vi "Init_core.vi"(8 "error in (no error)":errorcluster, 10 "VIRefIn":refnum<vi>, 11 "CtlReferences in":refnum<class "CtlReferences.lvclass">) -> (0 "error out":errorcluster, 3 "CtlReferences out":refnum<class "CtlReferences.lvclass">)   [LabVIEW 2020, in "CtlReferences.lvlib" / "CtlReferences.lvclass"]
uses:
  CtlReferences.lvclass
  CtlReferences.lvclass/CtlReferences.ctl
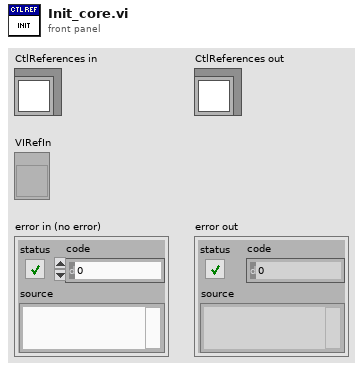
[diagram p1: front panel]
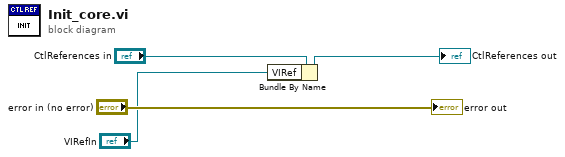
[diagram p0: block diagram]
diagram:
  n1 = Bundle By Name(cluster="CtlReferences in", "VIRef"="VIRefIn") -> (→"CtlReferences out":refnum<class "CtlReferences.lvclass">)
  "error out" <- "error in (no error)"
